vi "ZAlign_FilterAndSortConPane.vi"(7 "FilterCtrls[]":refnum<vi>[](array[refnum]), 8 "error in (no error)":errorcluster, 10 "TermBnds[]":T1[](array[typedef]), 11 "Ctrls[]":refnum<vi>[](array[refnum])) -> (0 "error out":errorcluster, 3 "Ctrls[]out":refnum<vi>[](array[refnum]) caption="Array")   [LabVIEW 2014, in "ZAlign.lvlib"]
doc: "ZAlign.lvlib:ZAlign_FilterAndSortConPane.vi\n----------------------------------------------\nFileter and sort Connector Pane\n\nInputs:\n---------------------\n- error in (no error) : Cluster; \n- TermBnds[] : 1DArrayOfCluster; \n- Ctrls[] : 1DArrayOfRefnum; \n\nOutputs:\n---------------------\n- error out : Cluster; \n- Array : 1DArrayOfRefnum; \n\n----------------------------------------------\n16/03/2015\nZühlke Engineering AG\nCH-8952 Schlieren\nwww.zuehlke.com"
uses:
  ZAlign.lvlib
  <vilib>/Utility/miscctls.llb/LVRectTypeDef.ctl
panel:
  # "Connector Pane"
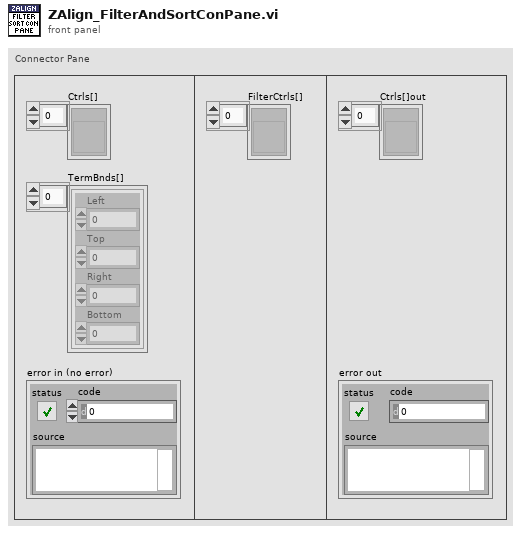
[diagram p1: front panel]
types:
  T1 = typedef "LVRectTypeDef.ctl" = cluster{"Left":i16, "Top":i16, "Right":i16, "Bottom":i16}
  T2 = typedef "LVPositionTypeDef.ctl" = cluster{"Left":i32, "Top":i32}
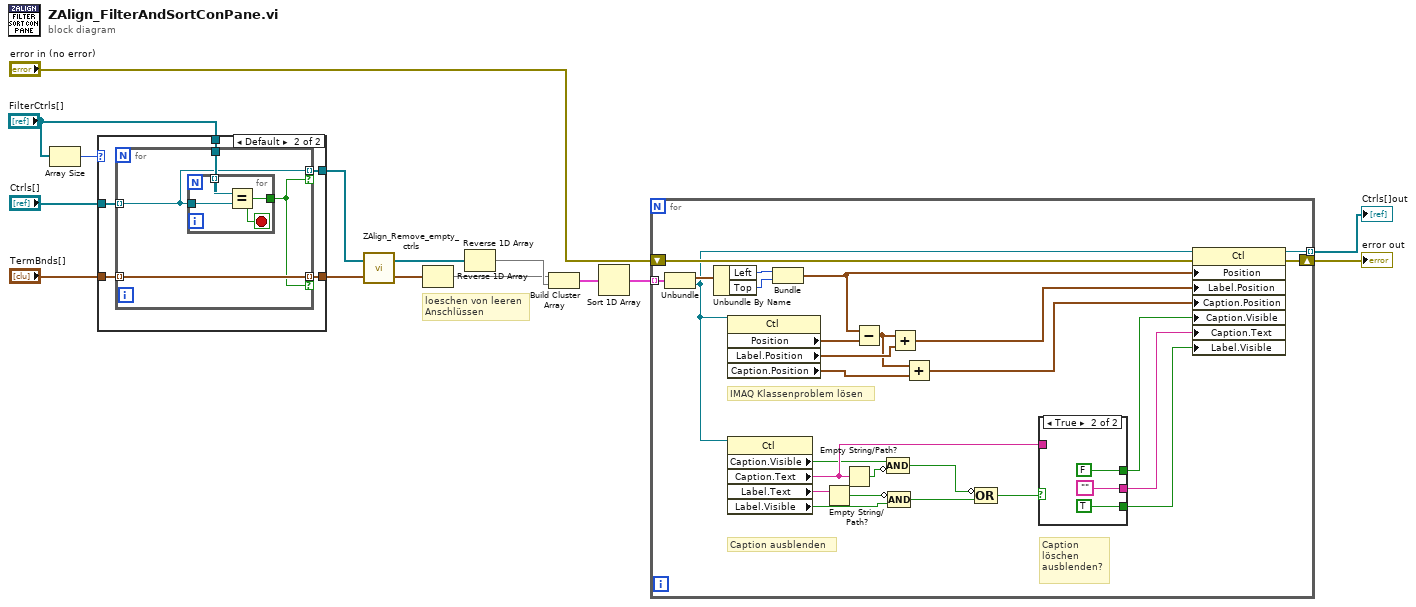
[diagram p0: block diagram]
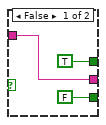
[diagram p3: hidden frame]
diagram:
  # "loeschen von leeren\nAnschlüssen"
  n1 = Array Size(array="FilterCtrls[]") -> (size(s)=w3:i32)
  n2 = case shown="Default" w3 {
    tunnel: "Ctrls[]" -> [w17 w22]
    tunnel: [w17 w21] -> w5
    tunnel: "FilterCtrls[]" -> [_ w20]
    tunnel: "TermBnds[]" -> [w16 w19]
    tunnel: [w16 w18] -> w1
    frame 0 {
    }
    frame Default {
      n3 = for {
        tunnel: w22 -> [w25] mode=indexing
        tunnel: w20 -> [w26]
        tunnel: [w25] -> w21 mode=indexing if=w23
        tunnel: w19 -> [w24] mode=indexing
        tunnel: [w24] -> w18 mode=indexing if=w23
        n4 = for {
          tunnel: w25 -> [w29]
          tunnel: w26 -> [w28] mode=indexing
          tunnel: [w27] -> w23
          stop <- w27 stop-if-true
          n5 = Equal?(x=w28, y=w29) -> (x = y?=w27:bool)
        }
      }
    }
  }
  n6 = call "ZAlign_Remove_empty_ctrls.vi"("TermBnds[]"=w1, "Controls in"=w5) -> ("Control locations"=w10:T1[], "Controls out"=w9:refnum<vi>[])
  n7 = Reverse 1D Array(array=w10) -> (reversed array=w12:T1[])
  n8 = Reverse 1D Array(array=w9) -> (reversed array=w13:refnum<vi>[])
  n9 = Build Cluster Array(w12, w13) -> (w14:cluster{"Rectangle":T1, refnum<vi>}[])
  n10 = Sort 1D Array(array=w14) -> (sorted array=w15:cluster{"Rectangle":T1, refnum<vi>}[])
  n11 = for {
    tunnel: [w55] -> w7 mode=indexing
    tunnel: w15 -> [w52] mode=indexing
    shift-right: [w54] -> w8
    shift-left: "error in (no error)" -> [w53]
    # "Caption \nlöschen\nausblenden?"
    # "Caption ausblenden"
    # "IMAQ Klassenproblem lösen"
    n12 = Unbundle(w52) -> ("Rectangle"=w51:T1, w42:refnum<vi>)
    n13 = Unbundle By Name(w51) -> ("Left"=w50:i16, "Top"=w56:i16)
    n14 = property class="Ctl"(reference=w42) -> ("Position"=w48:T2, "Label.Position"=w47:T2, "Caption.Position"=w44:T2)  [unwired: 1 in, 2 out]
    n15 = property class="Ctl"(reference=w42) -> ("Caption.Visible"=w36:bool, "Caption.Text"=w38:string, "Label.Text"=w41:string, "Label.Visible"=w32:bool)  [unwired: 1 in, 2 out]
    n16 = Bundle("Left"=w50, "Top"=w56) -> (w49:cluster{"Left":i16, "Top":i16})  [unwired: 1 in]
    n17 = Empty String/Path?(string/path=w41) -> (empty?=w33:bool)
    n18 = Empty String/Path?(string/path=w38) -> (empty?=w35:bool)
    n19 = Subtract(x=w49, y=w48) -> (x-y=w45:T2)
    n20 = Compound Arithmetic op=AND(w36, invert w35) -> (w30:bool)
    n21 = Compound Arithmetic op=AND(invert w33, w32) -> (w31:bool)
    n22 = Add(x=w45, y=w47) -> (x+y=w46:T2)
    n23 = Add(x=w45, y=w44) -> (x+y=w43:T2)
    n24 = Compound Arithmetic op=OR(invert w30, w31) -> (w34:bool)
    n25 = case shown="True" w34 {
      tunnel: [TRUE ("Caption.Visible") FALSE ("Caption.Visible")] -> w40
      tunnel: [w58 ""] -> w39
      tunnel: w38 -> [w58 _]
      tunnel: [FALSE ("Caption.Visible") TRUE ("Caption.Visible")] -> w37
      frame False {
      }
      frame True {
      }
    }
    n26 = property class="Ctl"(reference=w42, error in=w53, "Position"=w49, "Label.Position"=w46, "Caption.Position"=w43, "Caption.Visible"=w40, "Caption.Text"=w39, "Label.Visible"=w37) -> (reference out=w55:refnum<vi>, error out=w54:errorcluster)
  }
  "error out" <- w8
  "Ctrls[]out" <- w7
